vi "basic - VL Receive 2 VL.vi"() -> ()   [LabVIEW 2020]
uses:
  src/_polimorphicInstances/session/Fdx Close Session (Port).vi
  src/AIM664LV.lvlib
  src/_polimorphicInstances/udpPort/Fdx Create UDP Port (RX-CommPort).vi
  src/_polimorphicInstances/control/Fdx Stop (Rx).vi
  src/_polimorphicInstances/session/Fdx Create Session (Rx-VL-Oriented).vi
  src/bsp/AFDX_Receive/Fdx Create Rx VL.vi
  src/_polimorphicInstances/control/Fdx Start (Rx).vi
  src/_controls/comm_computedMAC-IP.ctl
  src/_controls/comm_verification_rx.ctl
  src/_controls/comm_udp_rx.ctl
panel:
  out "MsgCount 2":u32
  out "MsgErrorCount 2":u32
  out "MsgErrorCount":u32
  out "MsgCount":u32
  out "MsgRead 2":u32
  out "MsgRead":u32
  out "computedAddresses 2":T1 {"MACsrc" format="%.0x"}
  in  "CommPort Config 2":T2={"PortType"=enum."FDX_UDP_SAMPLING", "SubVIId"=1, "domainID"=1, "sideID"=1, "locationID"=1, "partitionID"=1, "UdpSrcPort"=12345, "UdpDstPort"=12346, "UdpNumBufMessages"=0, "UdpMaxMessageSize"=1000, "UdpSamplingRate"=128} {"partitionID" format="%.0b"}
  out "Data 2":u8[](array[numeric])
  in  "PortMap":u32
  out "Data":u8[](array[numeric])
  in  "CommPort Config 1":T2={"PortType"=enum."FDX_UDP_SAMPLING", "SubVIId"=1, "domainID"=1, "sideID"=1, "locationID"=1, "partitionID"=1, "UdpSrcPort"=12345, "UdpDstPort"=12346, "UdpNumBufMessages"=0, "UdpMaxMessageSize"=1000, "UdpSamplingRate"=128} {"partitionID" format="%.0b"}
  in  "VL Config":T3={"VlId"=60, "VLRange"=1, "VerificationMode"=0, "Bag"=0, "Jitter"=0, "MaxFrameLength"=0, "MaxSkew"=0, "VLBufSize"=32768, "FilterMode"=0, "FilterPosition"=0, "Padding"=0, "FilterMask"=0, "FilterData"=0, "MinFrameLength"=0} {"FilterMode" items=["FDX_RX_VL_FLT_DIS", "FDX_RX_VL_FLT_ENA ", "FDX_RX_VL_FLT_ENA_INV"]; "MaxFrameLength" format="%.0x"; "VerificationMode" items=["FDX_RX_VL_CHECK_ENA_DEFAULT"=65535, "FDX_RX_VL_CHECK_REDMAM"=16, "DX_RX_VL_CHECK_TRAFIC"=8, "FDX_RX_VL_CHECK_FRAMESIZE"=4, "FDX_RX_VL_CHECK_SNINTEG"=2, "FDX_RX_VL_CHECK_INVPAC"=1, "FDX_RX_VL_CHECK_DISA"=0]}
  in  "DefaultPayloadMode (Full)":u32(ring) items=["FDX_PAYLOAD_FULL", "FDX_PAYLOAD_IP_EXT", "FDX_PAYLOAD_IP", "FDX_PAYLOAD_MAC"]
  out "read time uS":cluster{u32, u32}(graph)
  in  "Port":u32=1
  in  "Board":u32
  out "current time":timestamp
  out "current irig time":T4={"SignOut"=-1509901600, "DayOut"=16, "HourOut"=8, "MinOut"=7, "SecondOut"=53, "MilliSecOut"=368, "MicroSecOut"=508, "NanoSecOut"=600, "InfoOut"=0, "Mode"=3}
  out "computedAddresses 1":T1 {"MACsrc" format="%.0x"}
  in  "stop":bool
  out "PortInitOut":T5 {"PortConfig" items=["FDX_SINGLE", "FDX_REDUNDANT"]}
  out "error out":errorcluster
  # "ARINC 664 - Receiving through VL (Virtual Link)"
  # "Overview: Setup the board to transmit package as raw frames.\nRequirement: One AIM ARINC-664 board with installed AIM ARINC 664 BSP.\nRestrictions: None.\nInstruction:\n1. Select the Board ID (0 if you have only one board in your system) and the port number. If you want to validate between two ports in one device, you can use tx board and Rx Board\n2. Run the VI.\n3. See the result in Current IRIG Time"
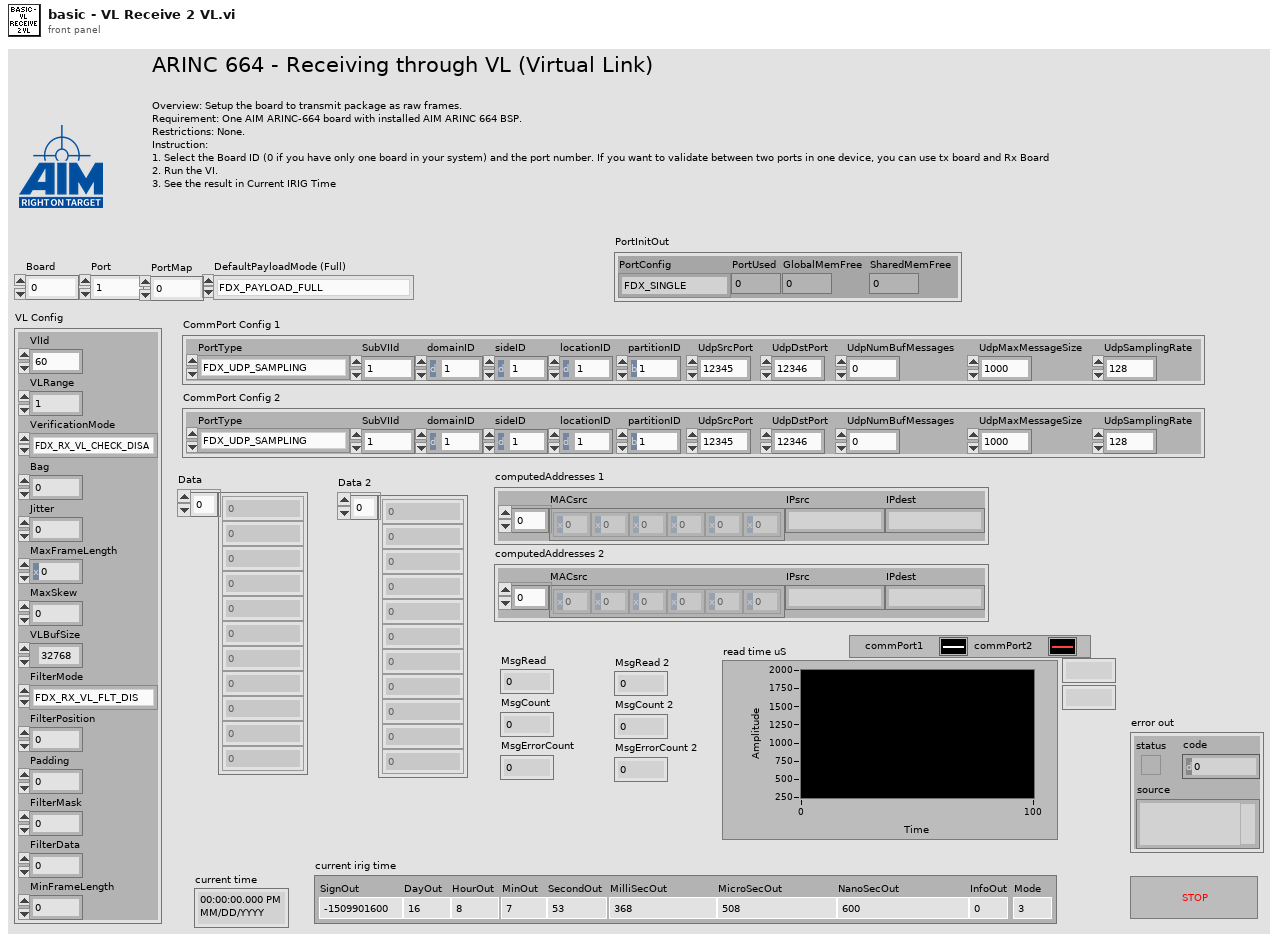
[diagram p1: front panel]
types:
  T1 = typedef "AIM664LV.lvlib/comm_computedMAC-IP.ctl" = cluster{"MACsrc":u8[], "IPsrc":string, "IPdest":string}
  T2 = typedef "AIM664LV.lvlib/comm_udp_rx.ctl" = cluster{"PortType":enum16{"FDX_UDP_SAMPLING", "FDX_UDP_QUEUING"}, "SubVIId":u32, "domainID":u8, "sideID":u8, "locationID":u8, "partitionID":u8, "UdpSrcPort":u16, "UdpDstPort":u16, "UdpNumBufMessages":u32, "UdpMaxMessageSize":u32, "UdpSamplingRate":u32}
  T3 = typedef "AIM664LV.lvlib/comm_verification_rx.ctl" = cluster{"VlId":u16, "VLRange":u32, "VerificationMode":u32, "Bag":u32, "Jitter":u32, "MaxFrameLength":u32, "MaxSkew":u32, "VLBufSize":u32, "FilterMode":u32, "FilterPosition":u32, "Padding":u32, "FilterMask":u32, "FilterData":u32, "MinFrameLength":u32}
  T4 = cluster{"SignOut":i32, "DayOut":u32, "HourOut":u32, "MinOut":u32, "SecondOut":u32, "MilliSecOut":u32, "MicroSecOut":u32, "NanoSecOut":u32, "InfoOut":u32, "Mode":u32}
  T5 = cluster{"PortConfig":u32, "PortUsed":u32, "GlobalMemFree":u32, "SharedMemFree":u32}
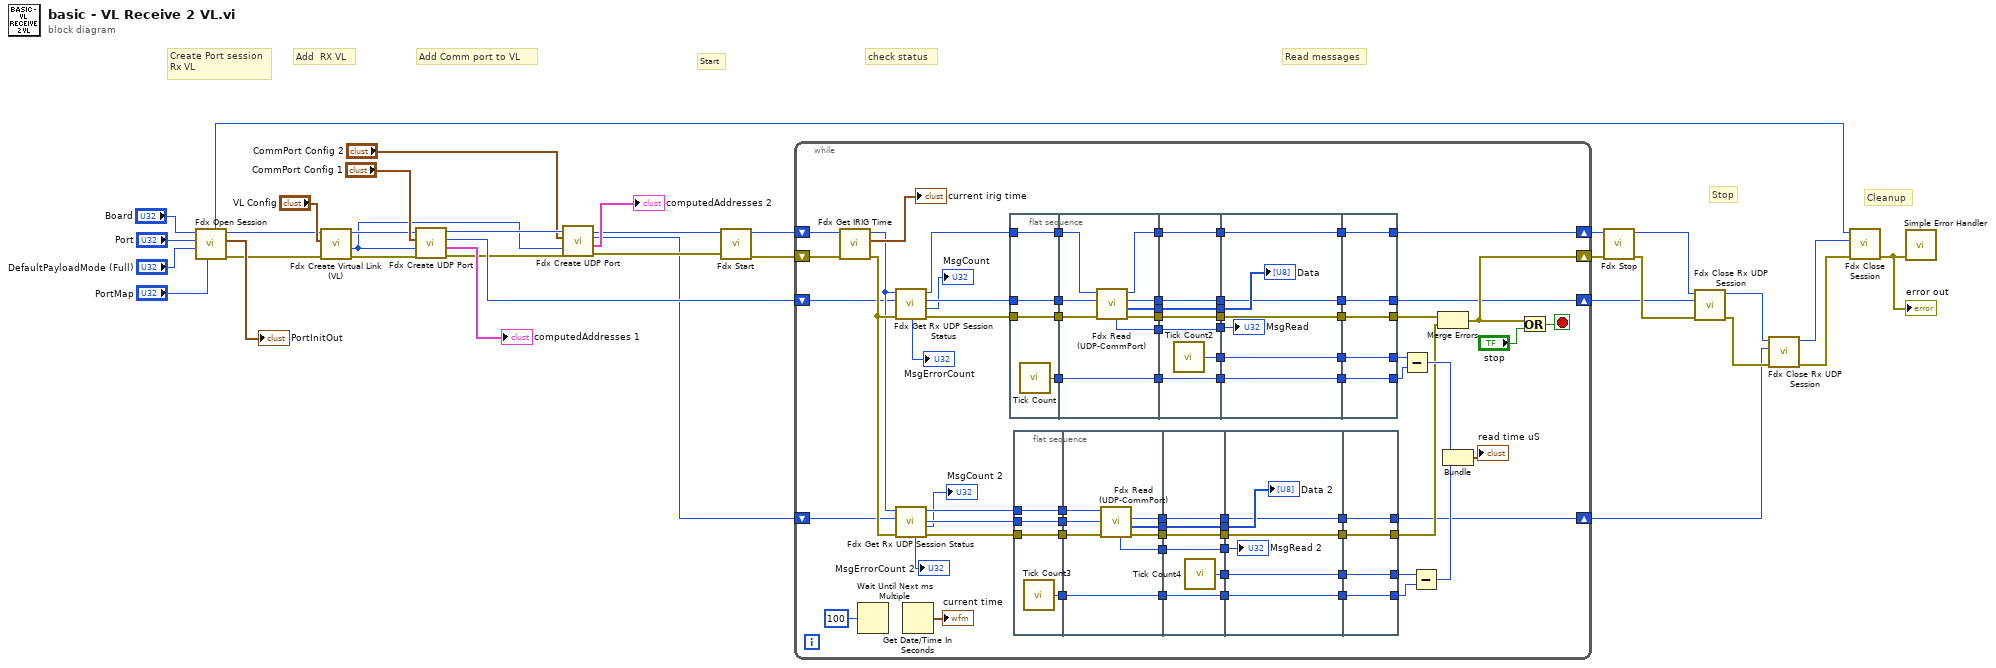
[diagram p0: block diagram]
diagram:
  # "Cleanup"
  # "Stop"
  # "Read messages"
  # "check status"
  # "Start"
  # "Add Comm port to VL"
  # "Add  RX VL"
  # "Create Port session\nRx VL"
  n1 = call-poly "Fdx Open Session.vi"("PortMap"="PortMap", "DefaultPayloadMode (Full)"="DefaultPayloadMode (Full)", "port"="Port", "board"="Board") -> ("error out"=w23:errorcluster, "PortInitOut"=→"PortInitOut":T5, "InstrumentHandle_port out"=w24:u32, "InstrumentHandle_board out"=w4:u32)  [unwired: 2 in, 2 out]
  n2 = call-poly "Fdx Create Virtual Link (VL).vi"("error in (no error)"=w23, "VL Config"="VL Config", "InstrumentHandle_port in"=w24) -> ("error out"=w26:errorcluster, "VlId"=w13:u16, "InstrumentHandle_port out"=w25:u32)  [unwired: 6 in]
  n3 = call-poly "Fdx Create UDP Port.vi"("error in (no error)"=w26, "VlId"=w13, "CommPort Config"="CommPort Config 1", "port handle in"=w25) -> ("error out"=w16:errorcluster, "computedAddresses"=→"computedAddresses 1":T1, "commPort handle out"=w20:u32, "port handle out"=w15:u32)  [unwired: 4 in]
  n4 = call-poly "Fdx Create UDP Port.vi"("error in (no error)"=w16, "VlId"=w13, "CommPort Config"="CommPort Config 2", "port handle in"=w15) -> ("error out"=w11:errorcluster, "computedAddresses"=→"computedAddresses 2":T1, "commPort handle out"=w5:u32, "port handle out"=w10:u32)  [unwired: 4 in]
  n5 = call-poly "Fdx Start.vi"("error in (no error)"=w11, "InstrumentHandle_port in"=w10) -> ("error out"=w34:errorcluster, "InstrumentHandle_port out"=w33:u32)  [unwired: 8 in]
  n6 = while {
    shift-right: [w91] -> w35
    shift-left: w33 -> [w107]
    shift-right: [w61] -> w21
    shift-left: w34 -> [w106]
    shift-right: [w39] -> w2
    shift-left: w20 -> [w48]
    shift-right: [w43] -> w3
    shift-left: w5 -> [w49]
    stop <- w109 stop-if-true
    n7 = call "Fdx Get IRIG Time.vi"("error in (no error)"=w106, "InstrumentHandle_board in"=w107) -> ("error out"=w54:errorcluster, "Curent Irig Time"=→"current irig time":T4, "InstrumentHandle_board out"=w50:u32)  [unwired: 7 in]
    n8 = Wait Until Next ms Multiple(millisecond multiple=u32 100) -> ()  [unwired: 1 out]
    n9 = call "Fdx Get Rx UDP Session Status.vi"("error in (no error)"=w54, "UdpHandle in"=w48, "InstrumentHandle_port in"=w50) -> ("error out"=w55:errorcluster, "MsgCount"=→"MsgCount":u32, "UdpHandle out"=w56:u32, "InstrumentHandle_port out"=w57:u32, "MsgErrorCount"=→"MsgErrorCount":u32)  [unwired: 4 in]
    n10 = call "Fdx Get Rx UDP Session Status.vi"("error in (no error)"=w54, "UdpHandle in"=w49, "InstrumentHandle_port in"=w50) -> ("error out"=w53:errorcluster, "MsgCount"=→"MsgCount 2":u32, "UdpHandle out"=w52:u32, "InstrumentHandle_port out"=w51:u32, "MsgErrorCount"=→"MsgErrorCount 2":u32)  [unwired: 4 in]
    n11 = Get Date/Time In Seconds() -> (seconds since 1Jan1904=→"current time":timestamp)
    n12 = flat-sequence {
      tunnel: w55 -> [w142]
      tunnel: [w142] -> w100
      tunnel: [w141] -> w99
      tunnel: w57 -> [w140]
      tunnel: [w140] -> w92
      tunnel: w56 -> [w139]
      tunnel: [w139] -> w86
      tunnel: w100 -> [w150]
      tunnel: [w149] -> w98
      tunnel: w99 -> [w151]
      tunnel: [w151] -> w96
      tunnel: w92 -> [w148]
      tunnel: [w147] -> w88
      tunnel: w86 -> [w146]
      tunnel: [w145] -> w84
      tunnel: [w144] -> w66
      tunnel: [w143] -> w36
      tunnel: w98 -> [w158]
      tunnel: [w158] -> w97
      tunnel: w96 -> [w157]
      tunnel: [w157] -> w95
      tunnel: [w156] -> w93
      tunnel: [w155] -> w89
      tunnel: w88 -> [w155]
      tunnel: [w154] -> w85
      tunnel: w84 -> [w154]
      tunnel: [w153] -> w67
      tunnel: w66 -> [w153]
      tunnel: [w152] -> w37
      tunnel: w36 -> [w152]
      tunnel: w97 -> [w162]
      tunnel: w95 -> [w165]
      tunnel: [w165] -> w102
      tunnel: [w164] -> w94
      tunnel: w93 -> [w164]
      tunnel: [w163] -> w90
      tunnel: w89 -> [w163]
      tunnel: [w162] -> w87
      tunnel: w85 -> [w161]
      tunnel: w67 -> [w160]
      tunnel: [w159] -> w38
      tunnel: w37 -> [w159]
      tunnel: [w170] -> w103
      tunnel: w102 -> [w170]
      tunnel: [w169] -> w68
      tunnel: w94 -> [w169]
      tunnel: [w168] -> w91
      tunnel: w90 -> [w168]
      tunnel: [w167] -> w83
      tunnel: w87 -> [w167]
      tunnel: [w166] -> w39
      tunnel: w38 -> [w166]
      frame #0 {
        n13 = call "Tick Count"() -> ("Tick Count(uSec)"=w141:u32)
      }
      frame #1 {
        n14 = call "Fdx Read (UDP-CommPort).vi"("error in (no error)"=w150, "UdpHandle in"=w146, "InstrumentHandle_port in"=w148) -> ("error out"=w149:errorcluster, "Data"=w145:u8[], "UdpHandle out"=w143:u32, "InstrumentHandle_port out"=w147:u32, "MsgRead"=w144:u32)  [unwired: 4 in]
      }
      frame #2 {
        n15 = call "Tick Count2"() -> ("Tick Count(uSec)"=w156:u32)
      }
      frame #3 {
        "Data" <- w161
        "MsgRead" <- w160
      }
      frame #4 {
      }
    }
    n16 = flat-sequence {
      tunnel: w53 -> [w114]
      tunnel: [w114] -> w82
      tunnel: [w113] -> w81
      tunnel: w51 -> [w112]
      tunnel: [w112] -> w80
      tunnel: w52 -> [w111]
      tunnel: [w111] -> w79
      tunnel: w82 -> [w121]
      tunnel: [w120] -> w78
      tunnel: w81 -> [w122]
      tunnel: [w122] -> w77
      tunnel: w80 -> [w119]
      tunnel: w79 -> [w118]
      tunnel: [w117] -> w76
      tunnel: [w116] -> w64
      tunnel: [w115] -> w40
      tunnel: w78 -> [w128]
      tunnel: [w128] -> w75
      tunnel: w77 -> [w127]
      tunnel: [w127] -> w74
      tunnel: [w126] -> w73
      tunnel: [w125] -> w72
      tunnel: w76 -> [w125]
      tunnel: [w124] -> w65
      tunnel: w64 -> [w124]
      tunnel: [w123] -> w41
      tunnel: w40 -> [w123]
      tunnel: w75 -> [w132]
      tunnel: w74 -> [w134]
      tunnel: [w134] -> w71
      tunnel: [w133] -> w70
      tunnel: w73 -> [w133]
      tunnel: [w132] -> w69
      tunnel: w72 -> [w131]
      tunnel: w65 -> [w130]
      tunnel: [w129] -> w42
      tunnel: w41 -> [w129]
      tunnel: [w138] -> w63
      tunnel: w71 -> [w138]
      tunnel: [w137] -> w62
      tunnel: w70 -> [w137]
      tunnel: [w136] -> w60
      tunnel: w69 -> [w136]
      tunnel: [w135] -> w43
      tunnel: w42 -> [w135]
      frame #0 {
        n17 = call "Tick Count3"() -> ("Tick Count(uSec)"=w113:u32)
      }
      frame #1 {
        n18 = call "Fdx Read (UDP-CommPort).vi"("error in (no error)"=w121, "UdpHandle in"=w118, "InstrumentHandle_port in"=w119) -> ("error out"=w120:errorcluster, "Data"=w117:u8[], "UdpHandle out"=w115:u32, "MsgRead"=w116:u32)  [unwired: 4 in, 1 out]
      }
      frame #2 {
        n19 = call "Tick Count4"() -> ("Tick Count(uSec)"=w126:u32)
      }
      frame #3 {
        "Data 2" <- w131
        "MsgRead 2" <- w130
      }
      frame #4 {
      }
    }
    n20 = Subtract(x=w68, y=w103) -> (x-y=w101:u32)
    n21 = Subtract(x=w62, y=w63) -> (x-y=w58:u32)
    n22 = Merge Errors(w83, w60) -> (w61:errorcluster)
    n23 = Bundle(w101, w58) -> (→"read time uS":cluster{u32, u32})  [unwired: 1 in]
    n24 = Or(x=w61, y="stop") -> (x .or. y?=w109:bool)
  }
  n25 = call-poly "Fdx Stop.vi"("error in (no error)"=w21, "InstrumentHandle_port in"=w35) -> ("error out"=w32:errorcluster, "InstrumentHandle_port out"=w19:u32)  [unwired: 8 in]
  n26 = call "Fdx Close Rx UDP Session.vi"("error in (no error)"=w32, "UdpHandle in"=w2, "InstrumentHandle_port in"=w19) -> ("error out"=w9:errorcluster, "InstrumentHandle_port out"=w7:u32)  [unwired: 7 in]
  n27 = call "Fdx Close Rx UDP Session.vi"("error in (no error)"=w9, "UdpHandle in"=w3, "InstrumentHandle_port in"=w7) -> ("error out"=w8:errorcluster, "InstrumentHandle_port out"=w6:u32)  [unwired: 7 in]
  n28 = call-poly "Fdx Close Session.vi"("error in (no error)"=w8, "InstrumentHandle_port in"=w6, "InstrumentHandle_board in"=w4) -> ("error out"=w1:errorcluster)  [unwired: 8 in]
  "error out" <- w1
  n29 = call <vilib>:"Simple Error Handler.vi"("error in (no error)"=w1) -> ()  [unwired: 4 in, 5 out]
